vi "Global_Video_Frame_Number.vi"() -> ()   [LabVIEW 2015]
panel:
  in  "Video Frame Number":u32
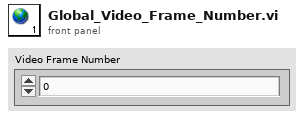
[diagram p1: front panel]
diagram:
